vi "RobotControlQueueIn.vi"() -> ()   [LabVIEW 2019]
panel:
  out "ModbusQue":refnum<queue>
  in  "SeverQue":refnum<queue>
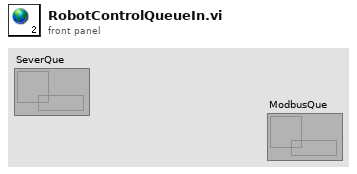
[diagram p1: front panel]
diagram:
